vi "Do Read.vi"(8 "error in (no error)":errorcluster, 10 "Interface":refnum<class "Interface.lvclass">, 11 "Section 2a in":refnum<class "Section 2a.lvclass">) -> (0 "error out":errorcluster, 2 "All Keys Found?":bool, 3 "Section 2a out":refnum<class "Section 2a.lvclass">)   [LabVIEW 2016, in "LVOOP Introduction.lvlib" / "Section 2a.lvclass"]
doc: "Read keys/value pairs from Interface.\n\nOverwriting dynamic dispatch VI."
uses:
  Section 2a.lvclass
  C:/User/Brand/LVP/VIP2012/Configuration/Classes/Section/Section.lvclass
  Configuration/Classes/Interface/Interface.lvclass
  Section 2a.lvclass/Section 2a.ctl
  Section 2/Section 2.lvclass
  Configuration/Classes/Section/Section.lvclass
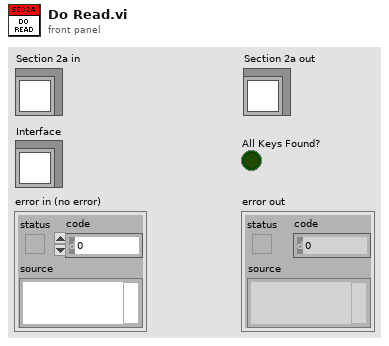
[diagram p1: front panel]
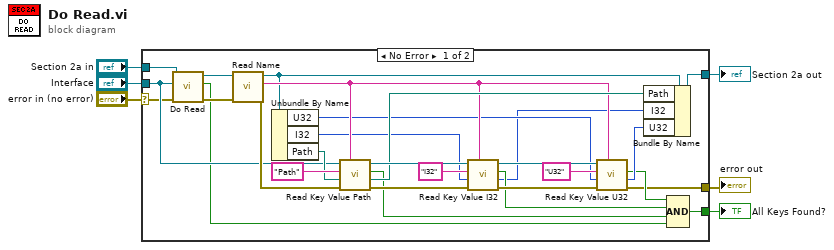
[diagram p0: block diagram]
diagram:
  n1 = case shown="No Error" "error in (no error)" {
    selector: "error in (no error)" -> [w9 w35]
    tunnel: "Interface" -> [w14 _]
    tunnel: "Section 2a in" -> [w13 w36]
    tunnel: [w12 w35] -> w4
    tunnel: [w11 w36] -> w3
    tunnel: [w10 _] -> w2
    frame No Error {
      n2 = call-parent "Do Read.vi"("error in (no error)"=w9, "Interface"=w14, "Section 2 in"=w13) -> ("error out"=w29:errorcluster, "All Keys Found?"=w7:bool, "Section 2 out"=w30:refnum<class "Section 2a.lvclass">)  [unwired: 6 in]
      n3 = call "Read Name.vi"("error in (no error)"=w29, "Section in"=w30) -> ("error out"=w28:errorcluster, "Name"=w24:string, "Section out"=w21:refnum<class "Section 2a.lvclass">)  [unwired: 7 in]
      n4 = Unbundle By Name(w21) -> ("U32"=w18:u32, "I32"=w19:i32, "Path"=w20:path)
      n5 = call-dynamic "Read Key Value Path.vi"("Section Name"=w24, "error in (no error)"=w28, "Default"=w20, "Key Name"="Path", "Interface in"=w14) -> ("error out"=w33:errorcluster, "Value"=w27:path, "found"=w15:bool, "Interface out"=w34:refnum<class "Interface.lvclass">)  [unwired: 3 in]
      n6 = call-dynamic "Read Key Value I32.vi"("Section Name"=w24, "error in (no error)"=w33, "Default"=w19, "Key Name"="I32", "Interface in"=w34) -> ("error out"=w31:errorcluster, "Value"=w8:i32, "found"=w16:bool, "Interface out"=w32:refnum<class "Interface.lvclass">)  [unwired: 3 in]
      n7 = call-dynamic "Read Key Value U32.vi"("Section Name"=w24, "error in (no error)"=w31, "Default"=w18, "Key Name"="U32", "Interface in"=w32) -> ("error out"=w12:errorcluster, "Value"=w26:u32, "found"=w17:bool)  [unwired: 3 in, 1 out]
      n8 = Bundle By Name(cluster=w21, "Path"=w27, "I32"=w8, "U32"=w26) -> (w11:refnum<class "Section 2a.lvclass">)
      n9 = Compound Arithmetic op=AND(w17, w16, w15, w7) -> (w10:bool)
    }
    frame Error {
    }
  }
  "error out" <- w4
  "Section 2a out" <- w3
  "All Keys Found?" <- w2
